vi "OriginalDigitizerLive - Copy.vi"() -> ()   [LabVIEW 2020]
doc: "Example Description:\nThis example demonstrates how to enable Time Interleaved Sampling with the NI 5772 adapter module to achieve a sampling rate of 1.6GS/s. This example continuously acquires records of analog input data from the NI 5772 adapter module. It allows you to select an AI channel, trigger type, and record size. This VI must be compiled before it is run. \n\nRunning the VI:\nThis VI must be run from the NI 5772 - Getting Started (Host).vi. Refer to the host VI documentation for steps regarding running and configuring the FPGA VI. \n\nExecution Steps:\nRefer to the Block Diagram of this VI for execution comments."
uses:
  Controls/AI Trigger Type.ctl
  Controls/Aquire State.ctl
  Controls/DownSampleState.ctl
  Controls/NeighbouringAvgStates.ctl
  <vilib>/Platform/TimedLoop/XDataNode/timing_clust.ctl
  <vilib>/Platform/TimedLoop/XDataNode/nitl_modes.ctl
  <vilib>/Platform/TimedLoop/XDataNode/wakeup.ctl
  <vilib>/rvi/Emulation/niFpgaGetClockAttributes.vi
  <vilib>/rvi/Emulation/niFpgaSctlEmulationGetInTimedLoop.vi
  <vilib>/rvi/Emulation/niFpgaEmulationReportErrorSimple.vi
  <vilib>/rvi/eio/common/nirviEmuTemplateMethod_errors.vi
  <vilib>/rvi/Emulation/niFpgaCriticalErrorInLSC.vi
  <vilib>/rvi/Emulation/niFpgaEmulationIsFPGAContextNoSignature.vi
  <vilib>/rvi/errors/niFpgaSetErrorForExecOnDevCompSimple.vi
  <vilib>/rvi/eio/common/nirviEmuReportErrorAndStop.vi
  <vilib>/rvi/DataTransferAndStorage/Container/Common/niFpgaContainerGetUniqueNameForEmu.vi
  <vilib>/rvi/FIFO/Fifo_Resource/nirvififoEmulationSetSize.vi
  <vilib>/rvi/FIFO/Fifo_Resource/nirviFifoEmulationQueueMgr.vi
  <instcachedir>/0/nirviFifoEmulationQueueMgr_E5CAEC123FF24DC58D834DCA3CDAA9B5.lvgen/nirviFifoEmulationQueueMgr_E5CAEC123FF24DC58D834DCA3CDAA9B5_000.vi
  <vilib>/Utility/error.llb/Clear Errors.vi
  <vilib>/rvi/FIFO/Fifo_Resource/nirvififoEmulationCreateLock.vi
  <vilib>/rvi/Emulation/niFpgaProcessEmulError.vi
  <vilib>/rvi/FIFO/Fifo_Resource/nirvififoEmulationObtainLock.vi
  <vilib>/rvi/FIFO/Fifo_Resource/nirvififoEmulationReleaseLock.vi
  <vilib>/rvi/occurrence/nirviWaitOnOccurrenceBase.vi
  <vilib>/rvi/errors/nirviReportUnexpectedCaseInternalError.vi
  <vilib>/rvi/errors/nirviReportUnexpectedCaseInternalError (U32).vi
  <vilib>/rvi/interface/RandomDataEmulation/niFpgaRandomDataHandleErrors.vi
  <vilib>/rvi/FIFO/Fifo_Resource/nirvififoEmulationDetermineInputValidOut.vi
  <vilib>/eio/EIONode/EIONode.xnode
  <vilib>/Platform/TimedLoop/XDataNode/XDataNode.xnode
  <vilib>/rvi/DataTransferAndStorage/Container/XNode/niFpgaContainer.xnode
  <vilib>/rvi/FIFO/Fifo_Resource/nirvififoEmulationRead.vi
  <vilib>/rvi/interface/RandomDataEmulation/nirviRandomDataFpgaReadWriteTemplate.vi
  <vilib>/rvi/FIFO/Fifo_Resource/nirvififoEmulationWrite.vi
  <vilib>/Platform/TimedLoop/XDataNode/XDNodeRunTimeDep.lvlib
  <instrlib>/_niInstr/Basic Elements/v1/FPGA/niInstr Basic Elements v1 FPGA.lvlib
panel:
  in  "Downsampling":T1
  in  "Trigger":bool=TRUE
  out "Acquire State":T2
  in  "Delay Cycles":u16=512 caption="Samples Per Trigger" min=1 step=1
  out "TS FIFO In Overflow?":bool caption="FIFO Overflow?"
  in  "Samples Per Trigger":u16=512 min=1 step=1
  in  "Arm Trigger":bool
  in  "User Command Commit":bool
  in  "User Command":u8
  out "User Command Idle":bool
  out "User Command Status":u8
  in  "User Data 0":u16
  in  "User Data 1":u8
  out "PLL Locked":bool
  out "User Error":bool
  out "Configured?":bool
  out "DMA FIFO Overflow?":bool caption="FIFO Overflow?"
  in  "Trigger Level":i16
  in  "Trigger Type":T3
  # "Resource Configuration"
  # "Refer to the Block Diagram of this VI for execution comments."
  # "For other instructions, select Help>>Show Context Help and move the cursor over the VI icon to display help for this VI."
  # "Analog Input"
  # "Clock Configuration"
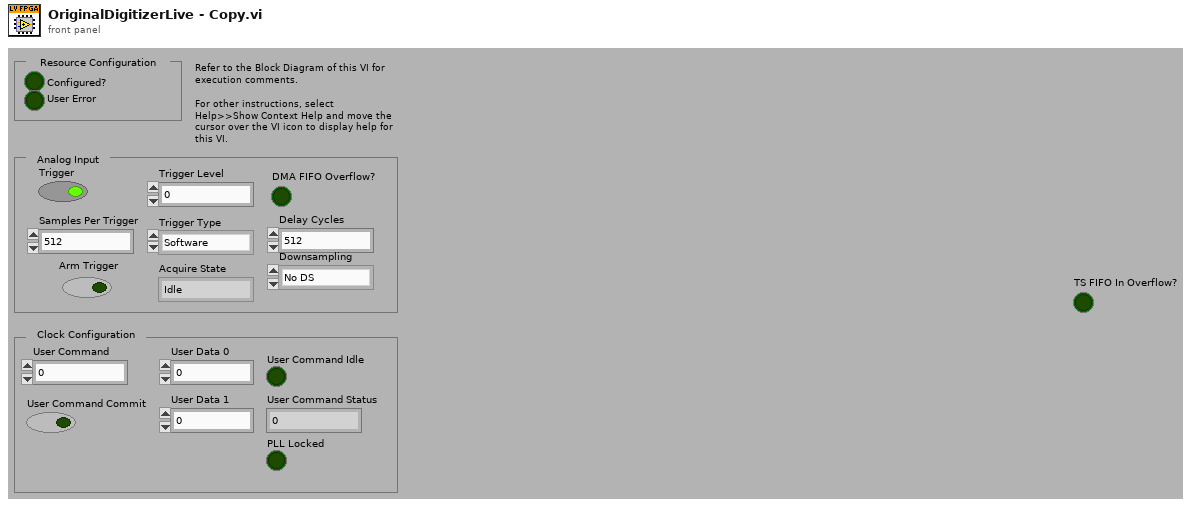
[diagram p1: front panel]
types:
  T1 = typedef "DownSampleState.ctl" = enum16{"No DS", "DS by 2", "DS by 4"}
  T2 = typedef "Aquire State.ctl" = enum8{"Idle", "Wait for Trigger", "AlignWave", "Hold Aquire", "Acquire", "WaitForWaveCompletion", "CheckAvg"}
  T3 = typedef "AI Trigger Type.ctl" = enum8{"Software", "Data Edge"}
  T4 = typedef "NeighbouringAvgStates.ctl" = enum16{"Idle", "Read_noDS", "Write1_noDS", "Write2_noDS", "Read1_DSby2", "Read2_DSby2"}
  T5 = typedef "XDNodeRunTimeDep.lvlib/timing_clust.ctl" = cluster{"Expected End [f-1]":u64, "Actual End [f-1]":u64, "Finished Late? [f-1]":bool, "Expected End [i-1]":u64, "Actual End [i-1]":u64, "Finished Late? [i-1]":bool, "Expected Start [i]":u64, "Actual Start [i]":u64, "Expected Start [f]":u64, "Actual Start [f]":u64, "Source Name":string, "Structure Name":string, "Period":i64, "Deadline":i64, "Offset":i64, "Start":i64, "Priority":i32, "Timeout":i32, "Mode":T6, "Wakeup Reason":T7, "Error":errorcluster, "Source Type":string, "Secondary Source Type":string, "Global End Time":u64, "Global Start Time":u64, "Frame Duration":u64, "Iteration Duration":u64, "Assigned CPU":i32, "I/O Scan Engine Mode":u32}
  T6 = typedef "XDNodeRunTimeDep.lvlib/nitl_modes.ctl" = enum32{"No Change", "Process missed periods, maintain original phase", "Discard missed periods, maintain original phase", "Process missed periods, ignore original phase", "Discard missed periods, ignore original phase"}
  T7 = typedef "XDNodeRunTimeDep.lvlib/wakeup.ctl" = enum32{"Normal", "Aborted", "Asynchronous wakeup", "Timing source error", "Timed loop error", "Timeout"}
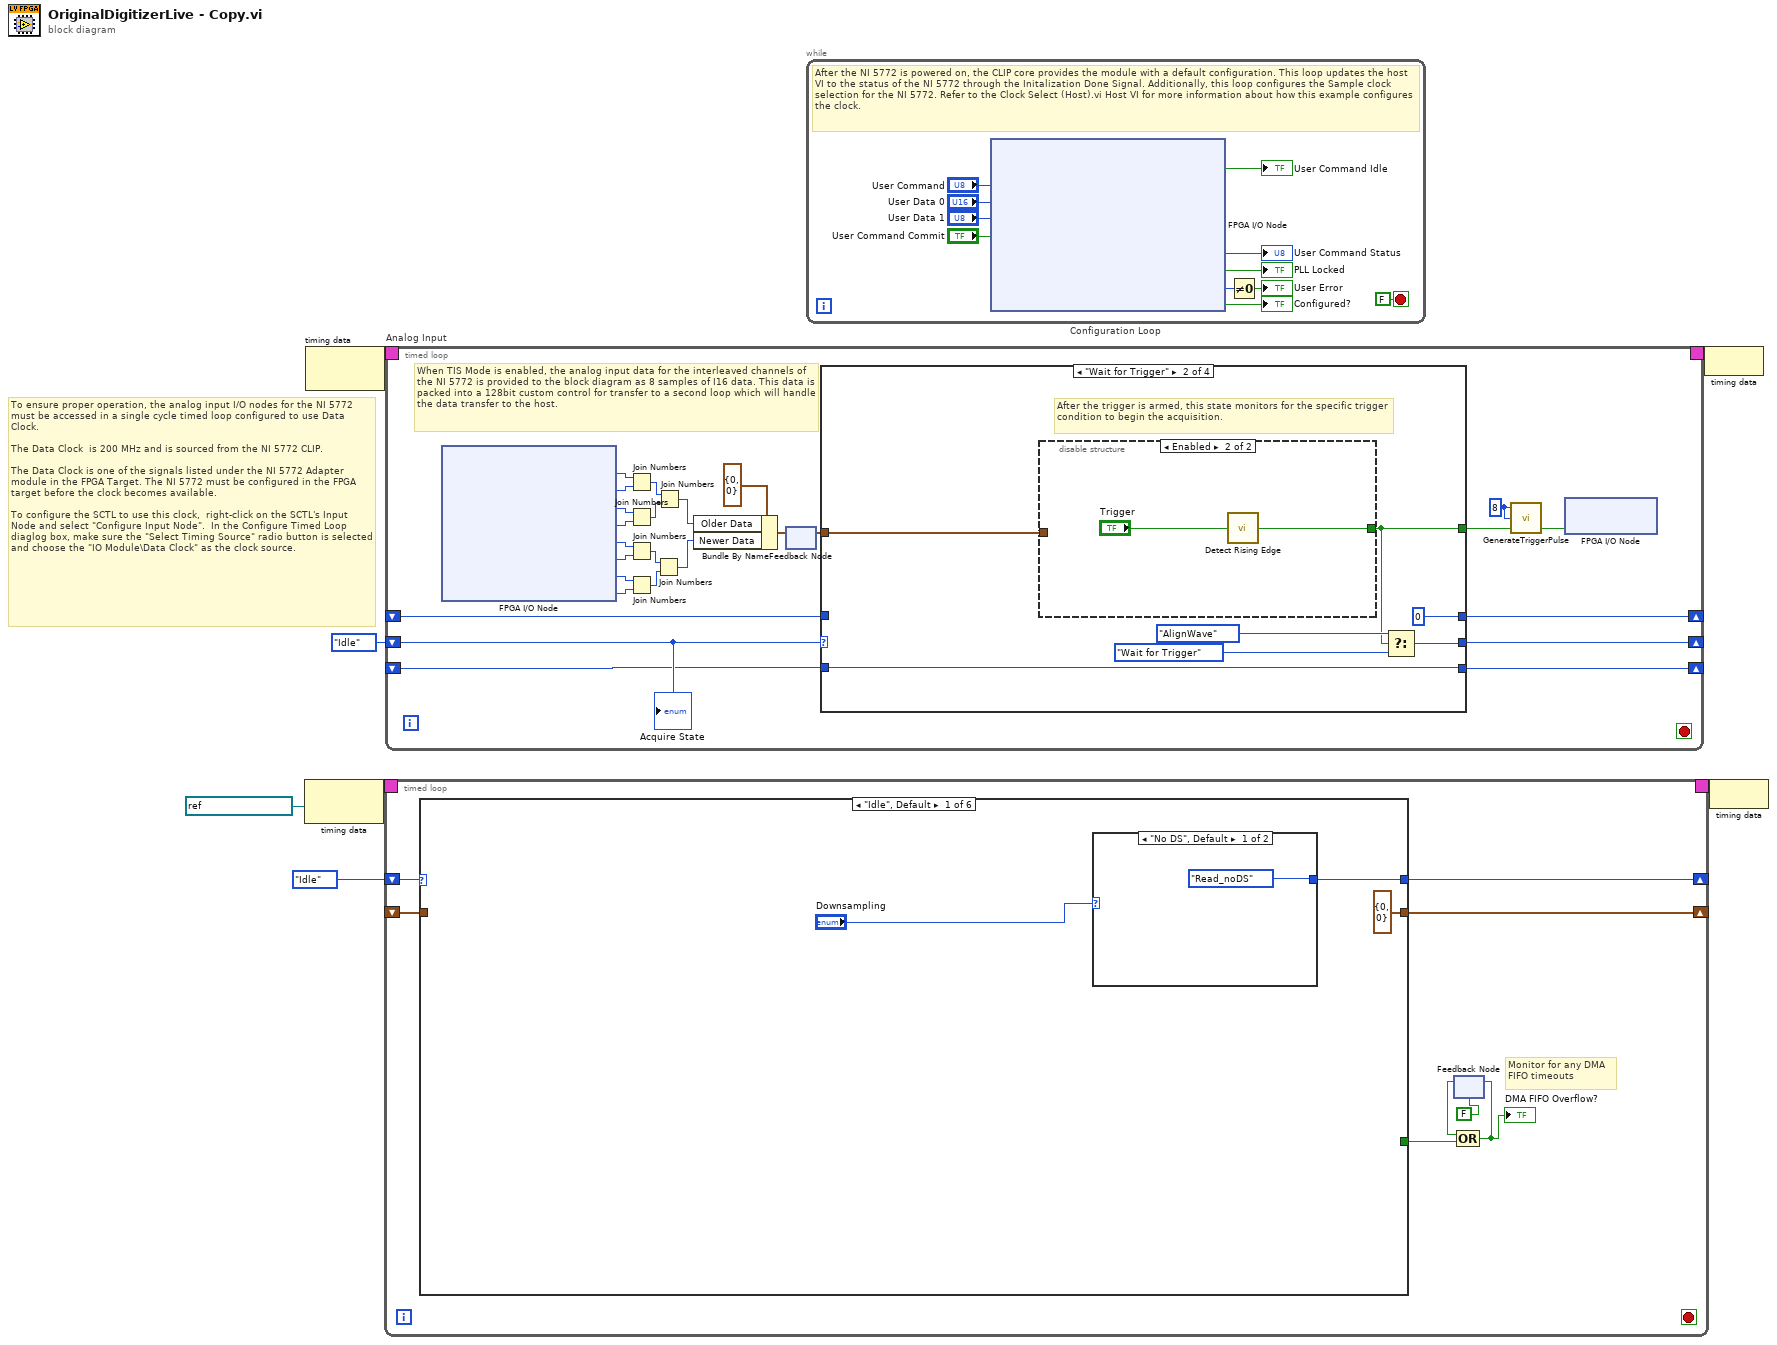
[diagram p0: block diagram]
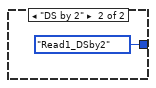
[diagram p2: hidden frame]
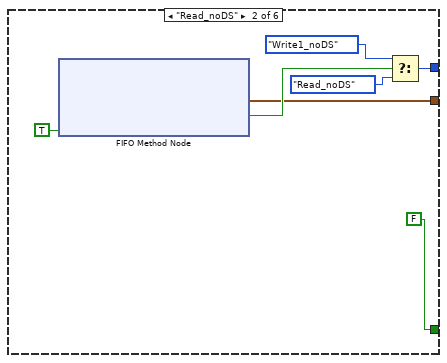
[diagram p3: hidden frame]
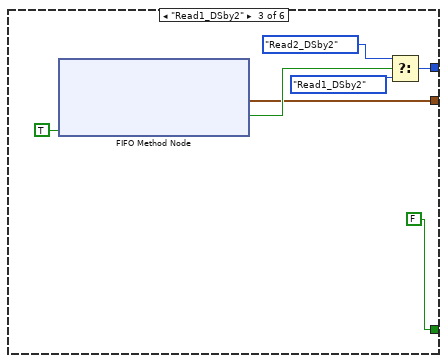
[diagram p4: hidden frame]
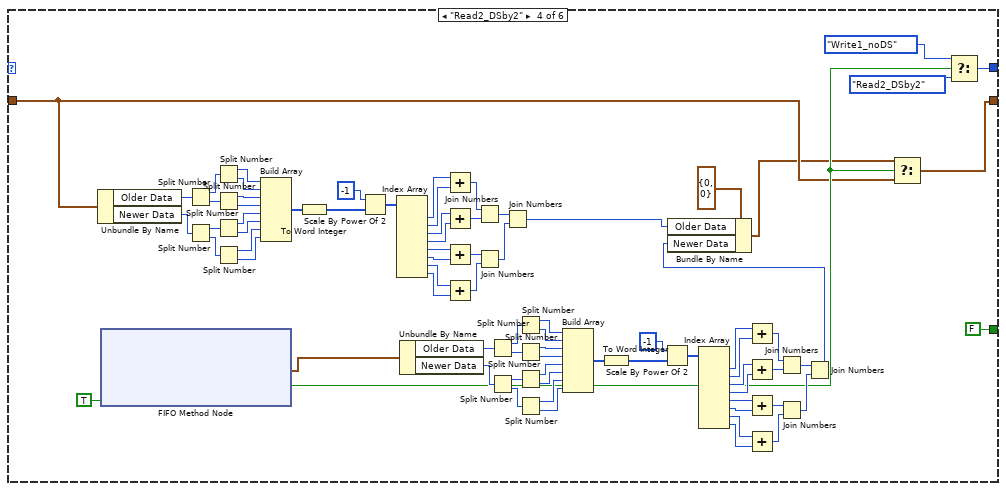
[diagram p5: hidden frame]
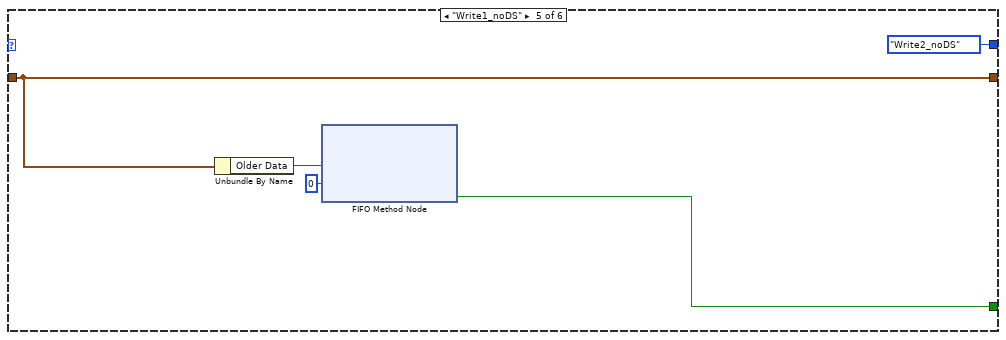
[diagram p6: hidden frame]
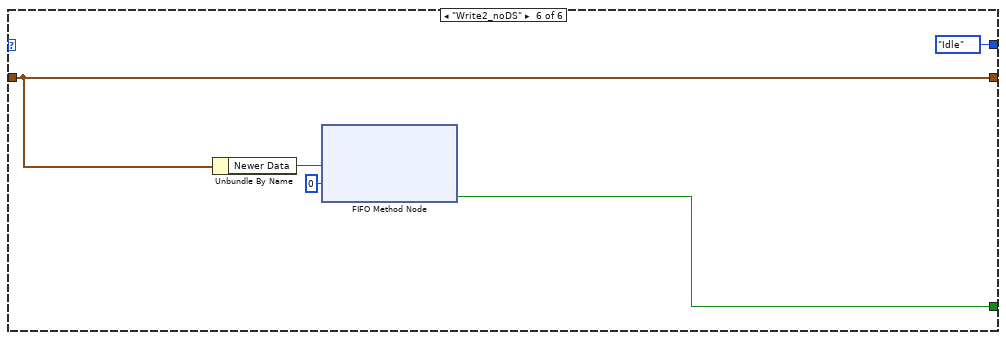
[diagram p7: hidden frame]
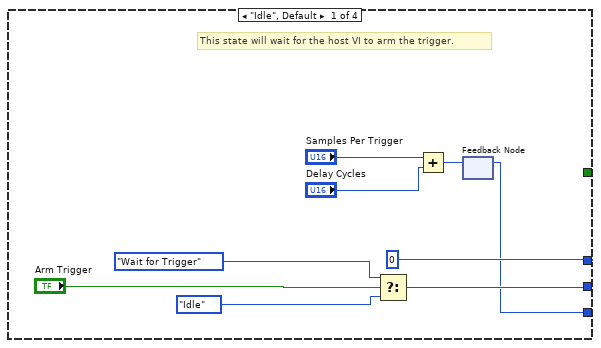
[diagram p8: hidden frame]
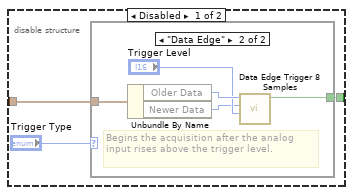
[diagram p9: hidden frame]
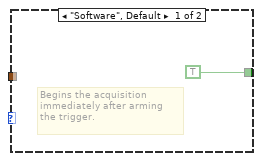
[diagram p10: hidden frame]
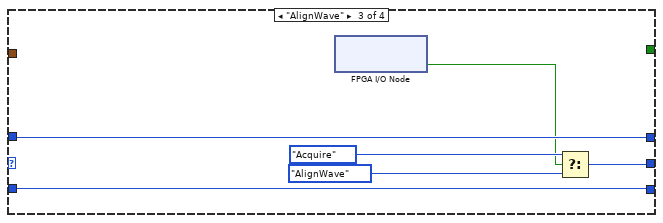
[diagram p11: hidden frame]
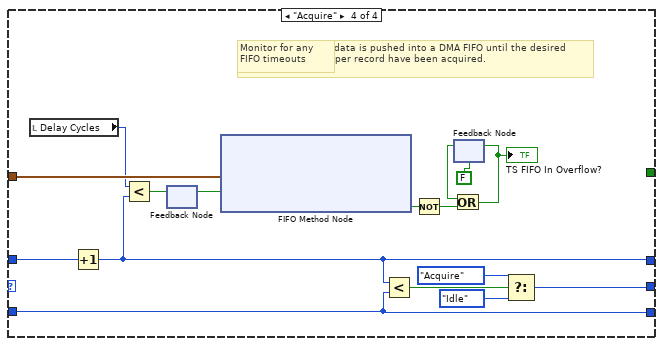
[diagram p12: hidden frame]
diagram:
  # "To ensure proper operation, the analog input I/O nodes for the NI 5772 must be accessed in a single cycle timed loop configured to use Data Clock. \n\nThe Data Clock  is 200 MHz and is sourced from the NI 5772 CLIP.\n\nThe Data Clock is one of the signals listed under the NI 5772 Adapter module in the FPGA Target. The NI 5772 must be configured in the FPGA target before the clock becomes available. \n\nTo configure the SCTL to use this clock,  right-click on the SCTL's Input Node and select \"Configure Input Node\".  In the Configure Timed Loop diaglog box, make sure the \"Select Timing Source\" radio button is selected and choose the \"IO Module\\Data Clock\" as the clock source."
  n1 = node-c288(refnum<k21> "200 MHz Clock" ("Source Name")) -> (w3:T5)
  n2 = node-c288() -> (w7:T5)  [unwired: 1 in]
  n3 = timed-loop {
    shift-right: [w14] -> _
    shift-left: NeighbouringAvgStates."Idle" -> [w15]
    shift-right: [w13] -> _
    shift-left: _ -> [w12]
    timing: w3 -> [_]
    timing-out: [_] -> w2
    stop <- _ stop-if-true
    # "Monitor for any DMA FIFO timeouts"
    n4 = case shown="\"Idle\", Default" w15 {
      tunnel: [w18 w27 w34 w111 NeighbouringAvgStates."Write2_noDS" NeighbouringAvgStates."Idle"] -> w14
      tunnel: [cluster{"Older Data":u64, "Newer Data":u64} {"Older Data"=0, "Newer Data"=0} ("Element") w23 w30 w36 w113 w118] -> w13
      tunnel: w12 -> [_ _ _ w37 w113 w118]
      tunnel: [_ FALSE ("Timed Out?") FALSE ("Timed Out?") FALSE ("Timed Out?") w114 w119] -> w9
      frame "Idle", Default {
        n5 = case shown="\"No DS\", Default" "Downsampling" {
          tunnel: [NeighbouringAvgStates."Read_noDS" NeighbouringAvgStates."Read1_DSby2"] -> w18
          frame "No DS", Default {
          }
          frame "DS by 2" {
          }
        }
      }
      frame "Read_noDS" {
        n6 = xnode ("FIFO Method Node")("Ready for Output"=TRUE) -> ("Element"=w23:cluster{"Older Data":u64, "Newer Data":u64}, "Output Valid"=w26:bool)  [unwired: 1 in, 1 out]
        n7 = Select(t=NeighbouringAvgStates."Write1_noDS", s=w26, f=NeighbouringAvgStates."Read_noDS") -> (s? t:f=w27:T4)
      }
      frame "Read1_DSby2" {
        n8 = xnode ("FIFO Method Node")("Ready for Output"=TRUE) -> ("Element"=w30:cluster{"Older Data":u64, "Newer Data":u64}, "Output Valid"=w33:bool)  [unwired: 1 in, 1 out]
        n9 = Select(t=NeighbouringAvgStates."Read2_DSby2", s=w33, f=NeighbouringAvgStates."Read1_DSby2") -> (s? t:f=w34:T4)
      }
      frame "Read2_DSby2" {
        n10 = Unbundle By Name(w37) -> ("Older Data"=w106:u64, "Newer Data"=w105:u64)
        n11 = xnode ("FIFO Method Node")("Ready for Output"=TRUE) -> ("Element"=w42:cluster{"Older Data":u64, "Newer Data":u64}, "Output Valid"=w38:bool)  [unwired: 1 in, 1 out]
        n12 = Split Number(x=w106) -> (hi(x)=w104:u32, lo(x)=w103:u32)
        n13 = Split Number(x=w105) -> (hi(x)=w102:u32, lo(x)=w101:u32)
        n14 = Split Number(x=w104) -> (hi(x)=w100:u16, lo(x)=w99:u16)
        n15 = Split Number(x=w103) -> (hi(x)=w98:u16, lo(x)=w97:u16)
        n16 = Split Number(x=w102) -> (hi(x)=w96:u16, lo(x)=w95:u16)
        n17 = Split Number(x=w101) -> (hi(x)=w94:u16, lo(x)=w93:u16)
        n18 = Build Array(w100, w99, w98, w97, w96, w95, w94, w93) -> (w92:u16[])
        n19 = To Word Integer(number=w92) -> (16bit integer=w90:i16[])
        n20 = Scale By Power Of 2(n=i16 -1, x=w90) -> (x*2^n=w89:i16[])
        n21 = Index Array(array=w89) -> (element #1=w87:i16, element #2=w88:i16, element #3=w86:i16, element #4=w85:i16, element #5=w84:i16, element #6=w83:i16, element #7=w82:i16, element #8=w81:i16)  [unwired: 8 in]
        n22 = Unbundle By Name(w42) -> ("Older Data"=w43:u64, "Newer Data"=w44:u64)
        n23 = Add(x=w87, y=w88) -> (x+y=w78:i16)
        n24 = Add(x=w86, y=w85) -> (x+y=w77:i16)
        n25 = Add(x=w84, y=w83) -> (x+y=w76:i16)
        n26 = Add(x=w82, y=w81) -> (x+y=w75:i16)
        n27 = Join Numbers(hi=w78, lo=w77) -> ((hi.lo)=w80:u32)
        n28 = Join Numbers(hi=w76, lo=w75) -> ((hi.lo)=w79:u32)
        n29 = Split Number(x=w43) -> (hi(x)=w45:u32, lo(x)=w46:u32)
        n30 = Split Number(x=w44) -> (hi(x)=w47:u32, lo(x)=w48:u32)
        n31 = Join Numbers(hi=w80, lo=w79) -> ((hi.lo)=w40:u64)
        n32 = Split Number(x=w45) -> (hi(x)=w49:u16, lo(x)=w50:u16)
        n33 = Split Number(x=w46) -> (hi(x)=w51:u16, lo(x)=w52:u16)
        n34 = Split Number(x=w47) -> (hi(x)=w53:u16, lo(x)=w54:u16)
        n35 = Split Number(x=w48) -> (hi(x)=w55:u16, lo(x)=w56:u16)
        n36 = Build Array(w49, w50, w51, w52, w53, w54, w55, w56) -> (w57:u16[])
        n37 = To Word Integer(number=w57) -> (16bit integer=w59:i16[])
        n38 = Scale By Power Of 2(n=i16 -1, x=w59) -> (x*2^n=w60:i16[])
        n39 = Index Array(array=w60) -> (element #1=w62:i16, element #2=w61:i16, element #3=w63:i16, element #4=w64:i16, element #5=w65:i16, element #6=w66:i16, element #7=w67:i16, element #8=w68:i16)  [unwired: 8 in]
        n40 = Add(x=w62, y=w61) -> (x+y=w71:i16)
        n41 = Add(x=w63, y=w64) -> (x+y=w72:i16)
        n42 = Add(x=w65, y=w66) -> (x+y=w73:i16)
        n43 = Add(x=w67, y=w68) -> (x+y=w74:i16)
        n44 = Join Numbers(hi=w71, lo=w72) -> ((hi.lo)=w69:u32)
        n45 = Join Numbers(hi=w73, lo=w74) -> ((hi.lo)=w70:u32)
        n46 = Join Numbers(hi=w69, lo=w70) -> ((hi.lo)=w39:u64)
        n47 = Bundle By Name(cluster=cluster{"Older Data":u64, "Newer Data":u64} {"Older Data"=0, "Newer Data"=0} ("Element"), "Older Data"=w40, "Newer Data"=w39) -> (w35:cluster{"Older Data":u64, "Newer Data":u64})
        n48 = Select(t=w35, s=w38, f=w37) -> (s? t:f=w36:cluster{"Older Data":u64, "Newer Data":u64})
        n49 = Select(t=NeighbouringAvgStates."Write1_noDS", s=w38, f=NeighbouringAvgStates."Read2_DSby2") -> (s? t:f=w111:T4)
      }
      frame "Write1_noDS" {
        n50 = Unbundle By Name(w113) -> ("Older Data"=w115:u64)
        n51 = xnode ("FIFO Method Node")("Element"=w115, "Timeout"=0) -> ("Timed Out?"=w114:bool)  [unwired: 1 in, 1 out]
      }
      frame "Write2_noDS" {
        n52 = Unbundle By Name(w118) -> ("Newer Data"=w120:u64)
        n53 = xnode ("FIFO Method Node")("Element"=w120, "Timeout"=0) -> ("Timed Out?"=w119:bool)  [unwired: 1 in, 1 out]
      }
    }
    n54 = feedback #1(FALSE) -> (w10:bool)
    n55 = Compound Arithmetic op=OR(w10, w9) -> (w11:bool)
    "DMA FIFO Overflow?" <- w11
    n56 = feedback-in #1(w11) -> ()
  }
  n57 = timed-loop "Analog Input" {
    timing: w7 -> [_]
    timing-out: [_] -> w6
    shift-right: [w148] -> _
    shift-left: Aquire_State."Idle" ("Acquire State") -> [w138]
    shift-right: [w149] -> _
    shift-left: _ -> [w139]
    shift-right: [w147] -> _
    shift-left: _ -> [w137]
    stop <- _ stop-if-true
    w125 = u16 8 ("Pulse Width On [cycles]")
    # "When TIS Mode is enabled, the analog input data for the interleaved channels of the NI 5772 is provided to the block diagram as 8 samples of I16 data. This data is packed into a 128bit custom control for transfer to a second loop which will handle the data transfer to the host."
    n58 = xnode "FPGA I/O Node"() -> ("IO Module\\AI 1 Data N-3"=w130:i16, "IO Module\\AI 0 Data N-3"=w129:i16, "IO Module\\AI 1 Data N-2"=w128:i16, "IO Module\\AI 0 Data N-2"=w127:i16, "IO Module\\AI 1 Data N-1"=w131:i16, "IO Module\\AI 0 Data N-1"=w132:i16, "IO Module\\AI 1 Data N"=w133:i16, "IO Module\\AI 0 Data N"=w134:i16)  [unwired: 8 in, 8 out]
    n59 = Join Numbers(hi=w130, lo=w129) -> ((hi.lo)=w142:u32)
    n60 = Join Numbers(hi=w128, lo=w127) -> ((hi.lo)=w144:u32)
    n61 = Join Numbers(hi=w131, lo=w132) -> ((hi.lo)=w143:u32)
    n62 = Join Numbers(hi=w133, lo=w134) -> ((hi.lo)=w145:u32)
    n63 = Join Numbers(hi=w143, lo=w145) -> ((hi.lo)=w135:u64)
    n64 = Join Numbers(hi=w142, lo=w144) -> ((hi.lo)=w136:u64)
    n65 = Bundle By Name(cluster=cluster{"Older Data":u64, "Newer Data":u64} {"Older Data"=0, "Newer Data"=0} ("Element"), "Older Data"=w136, "Newer Data"=w135) -> (w140:cluster{"Older Data":u64, "Newer Data":u64})
    n66 = feedback #2() -> (w146:cluster{"Older Data":u64, "Newer Data":u64})  [unwired: 1 in]
    n67 = feedback-in #2(w140) -> ()
    n68 = case shown="\"Wait for Trigger\"" w138 {
      tunnel: [u16 0 u16 0 w179 w190] -> w149
      tunnel: w139 -> [_ _ w179 w198]
      tunnel: [w155 w161 w180 w196] -> w148
      tunnel: [w151 w165 w178 w193] -> w147
      tunnel: w137 -> [_ w165 w178 w193]
      tunnel: w146 -> [_ w164 _ w192]
      tunnel: [_ w159 _ _] -> w124
      frame "Idle", Default {
        # "This state will wait for the host VI to arm the trigger."
        n69 = Select(t=Aquire_State."Wait for Trigger" ("Acquire State"), s="Arm Trigger", f=Aquire_State."Idle" ("Acquire State")) -> (s? t:f=w155:T2)
        n70 = Add(x="Samples Per Trigger", y="Delay Cycles") -> (x+y=w152:u16)
        n71 = feedback-in #3(w152) -> ()
        n72 = feedback #3() -> (w151:u16)  [unwired: 1 in]
      }
      frame "Wait for Trigger" {
        # "After the trigger is armed, this state monitors for the specific trigger condition to begin the acquisition."
        n73 = disable-structure shown="Enabled" {
          disable-tunnel: w164 -> [w167 _]
          disable-tunnel: [w166 w175] -> w159
          frame Disabled {
            n74 = case shown="\"Data Edge\"" "Trigger Type" {
              tunnel: w167 -> [_ w174]
              tunnel: [TRUE ("Trigger") w173] -> w166
              frame "Software", Default {
                # "Begins the acquisition immediately after arming the trigger."
              }
              frame "Data Edge" {
                # "Begins the acquisition after the analog input rises above the trigger level."
                n75 = Unbundle By Name(w174) -> ("Older Data"=w172:u64, "Newer Data"=w170:u64)
                n76 = call "Data Edge Trigger 8 Samples.vi"("Trigger Level"="Trigger Level", "Newer Data In"=w170, "Older Data In"=w172) -> ("Trigger"=w173:bool)  [unwired: 8 in]
              }
            }
          }
          frame Enabled {
            n77 = call <instrlib>:"Detect Rising Edge.vi"("signal"="Trigger") -> ("edge detected"=w175:bool)  [unwired: 14 in]
          }
        }
        n78 = Select(t=Aquire_State."AlignWave" ("Acquire State"), s=w159, f=Aquire_State."Wait for Trigger") -> (s? t:f=w161:T2)
      }
      frame "AlignWave" {
        n79 = xnode "FPGA I/O Node"() -> ("PXI_Trig0"=w177:bool)  [unwired: 1 in, 1 out]
        n80 = Select(t=Aquire_State."Acquire" ("Acquire State"), s=w177, f=Aquire_State."AlignWave") -> (s? t:f=w180:T2)
      }
      frame "Acquire" {
        # "Monitor for any  FIFO timeouts"
        # "While in this state, data is pushed into a DMA FIFO until the desired number of samples per record have been acquired."
        n81 = local read "Delay Cycles"() -> (w191:u16)
        n82 = Increment(x=w198) -> (x+1=w190:u16)
        n83 = Less?(x=w191, y=w190) -> (x < y?=w186:bool)
        n84 = feedback-in #4(w186) -> ()
        n85 = feedback #4() -> (w183:bool)  [unwired: 1 in]
        n86 = xnode ("FIFO Method Node")("Element"=w192, "Input Valid"=w183) -> ("Ready for Input"=w185:bool)  [unwired: 1 in, 1 out]
        n87 = Less?(x=w190, y=w193) -> (x < y?=w197:bool)
        n88 = Not(x=w185) -> (.not. x?=w184:bool)
        n89 = feedback #5(FALSE) -> (w187:bool)
        n90 = Or(x=w187, y=w184) -> (x .or. y?=w188:bool)
        "TS FIFO In Overflow?" <- w188
        n91 = feedback-in #5(w188) -> ()
        n92 = Select(t=Aquire_State."Acquire" ("Acquire State"), s=w197, f=Aquire_State."Idle" ("Acquire State")) -> (s? t:f=w196:T2)
      }
    }
    n93 = call "GenerateTriggerPulse.vi"("Trigger"=w124, "Pulse Width Off [cycles]"=w125, "Pulse Width On [cycles]"=w125) -> ("Out"=w126:bool)  [unwired: 2 out]
    n94 = xnode "FPGA I/O Node"("PXI_Trig1"=w126) -> ()  [unwired: 1 in, 1 out]
    "Acquire State" <- w138
  }
  n95 = while "Configuration Loop" {
    stop <- FALSE stop-if-true
    # "After the NI 5772 is powered on, the CLIP core provides the module with a default configuration. This loop updates the host VI to the status of the NI 5772 through the Initalization Done Signal. Additionally, this loop configures the Sample clock selection for the NI 5772. Refer to the Clock Select (Host).vi Host VI for more information about how this example configures the clock."
    n96 = xnode "FPGA I/O Node"("IO Module\\User Command"="User Command", "IO Module\\User Data 0"="User Data 0", "IO Module\\User Data 1"="User Data 1", "IO Module\\User Command Commit"="User Command Commit") -> ("IO Module\\User Command Idle"=→"User Command Idle":bool, "IO Module\\User Command Status"=→"User Command Status":u8, "IO Module\\PLL Locked"=→"PLL Locked":bool, "IO Module\\User Error"=w206:u8, "IO Module\\Initialization Done"=→"Configured?":bool)  [unwired: 9 in, 9 out]
    n97 = Not Equal To 0?(x=w206) -> (x != 0?=→"User Error":bool)
  }
  n98 = node-c288(w6) -> ()
  n99 = node-c288(w2) -> ()
